vi "Tree_Sync Symbols Handler_ACAF.vi"(7 "Action":T1, 8 "error in (no error)":errorcluster, 11 "Tree Ref Array":refnum<vi>[](array[refnum])) -> (0 "error out":errorcluster, 3 "Tree Ref Array Out":refnum<vi>[](array[refnum]))   [LabVIEW 2023]
doc: "Synchronize symbols and value across the three trees. Clicking on the main VI will select a symbol if none is selected. Clicking on a symbol will select or deselect the row. A tree value is maintained, which survives filtering on the tree.\n\nThis VI initializes the tree value to no selection on run."
uses:
  controls/action enum.ctl
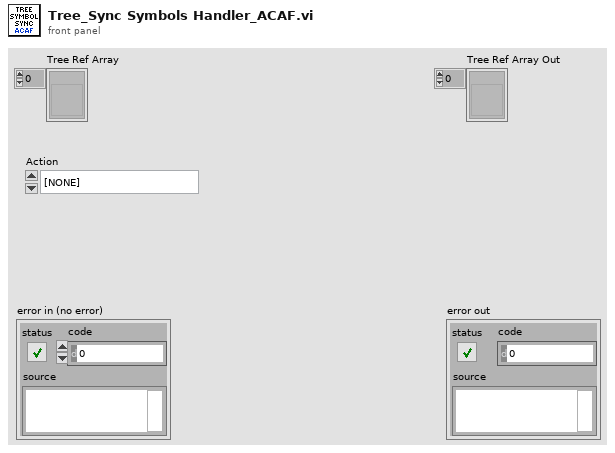
[diagram p1: front panel]
types:
  T1 = typedef "action enum.ctl" = enum16{"[NONE]", "APP_SEPARATOR", "Wire Bundle", "Wire Unbundle", "Terminal Unbundle", "Terminal Bundle", "Bundler Move Up", "Bundler Move Down", "Bundler Insert", "Bundler Remove", "Bundler Remove Unwired", "Bundler Reorder", "In Place Insert", "In Place Remove", "In Place Remove Unwired", "In Place Reorder", "Wire Properties", "Wire Method", "Terminal Properties", "Terminal Method", "Property Move Up", "Property Move Down", "Properties Insert", "Properties Remove", "Properties Remove Unwired", "Properties Reorder", "Method Change", "Class For Constant", "Class For Control", "Class For Node", "Class Name to Clipboard"}
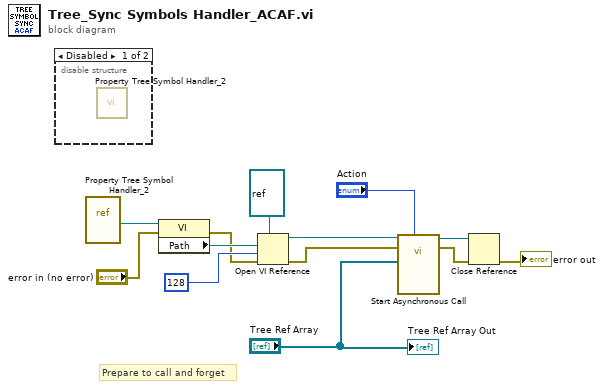
[diagram p0: block diagram]
diagram:
  # "Prepare to call and forget"
  n1 = disable-structure shown="Disabled" {
    frame Disabled {
      n2 = call "Property Tree Symbol Handler_2.vi"() -> ()  [unwired: 12 in]
    }
    frame Enabled {
    }
  }
  n3 = vi-ref "Property Tree Symbol Handler_2.vi"() -> (w13:refnum<vi>)
  n4 = property class="VI"(reference=w13, error in="error in (no error)") -> (error out=w3:errorcluster, "Path"=w9:path)  [unwired: 1 out]
  n5 = Open VI Reference(type specifier VI Refnum (for type only)=refnum<vi> refnum, vi path=w9, options=128, error in (no error)=w3) -> (vi reference=w4:refnum<vi>, error out=w8:errorcluster)  [unwired: 2 in]
  n6 = call-by-ref "Start Asynchronous Call"(reference=w4, error in=w8, "Save Action"="Action", "Tree refs"="Tree Ref Array") -> (reference out=w7:refnum<vi>, error out=w6:errorcluster)  [unwired: 10 in]
  n7 = Close Reference(reference=w7, error in (no error)=w6) -> (error out=→"error out":errorcluster)
  "Tree Ref Array Out" <- "Tree Ref Array"
